vi "Error UI.vi"() -> ()   [LabVIEW 2012]
uses:
  <vilib>/Platform/TimedLoop/XDataNode/timing_clust.ctl
  <vilib>/Platform/TimedLoop/XDataNode/nitl_modes.ctl
  <vilib>/Platform/TimedLoop/XDataNode/wakeup.ctl
  <vilib>/Platform/TimedLoop/XDataNode/XDataNode.xnode
  <vilib>/Platform/TimedLoop/XDataNode/XDNodeRunTimeDep.lvlib
panel:
  out "Error":bool
  out "OK":bool
  in  "stop?":bool
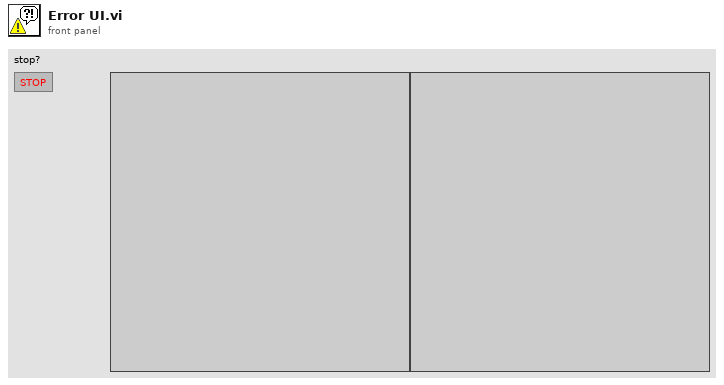
[diagram p1: front panel]
types:
  T1 = typedef "XDNodeRunTimeDep.lvlib/timing_clust.ctl" = cluster{"Expected End [f-1]":u64, "Actual End [f-1]":u64, "Finished Late? [f-1]":bool, "Expected End [i-1]":u64, "Actual End [i-1]":u64, "Finished Late? [i-1]":bool, "Expected Start [i]":u64, "Actual Start [i]":u64, "Expected Start [f]":u64, "Actual Start [f]":u64, "Source Name":string, "Structure Name":string, "Period":i64, "Deadline":i64, "Offset":i64, "Start":i64, "Priority":i32, "Timeout":i32, "Mode":T2, "Wakeup Reason":T3, "Error":errorcluster, "Source Type":string, "Secondary Source Type":string, "Global End Time":u64, "Global Start Time":u64, "Frame Duration":u64, "Iteration Duration":u64, "Assigned CPU":i32, "I/O Scan Engine Mode":u32}
  T2 = typedef "XDNodeRunTimeDep.lvlib/nitl_modes.ctl" = enum32{"No Change", "Process missed periods, maintain original phase", "Discard missed periods, maintain original phase", "Process missed periods, ignore original phase", "Discard missed periods, ignore original phase"}
  T3 = typedef "XDNodeRunTimeDep.lvlib/wakeup.ctl" = enum32{"Normal", "Aborted", "Asynchronous wakeup", "Timing source error", "Timed loop error", "Timeout"}
  T4 = enum16{"Idle", "Wiimote", "Joypad", "IGVC", "Avoide Objects", "Avoide Lines", "Path Planning", "Heading", "Waypoint"}
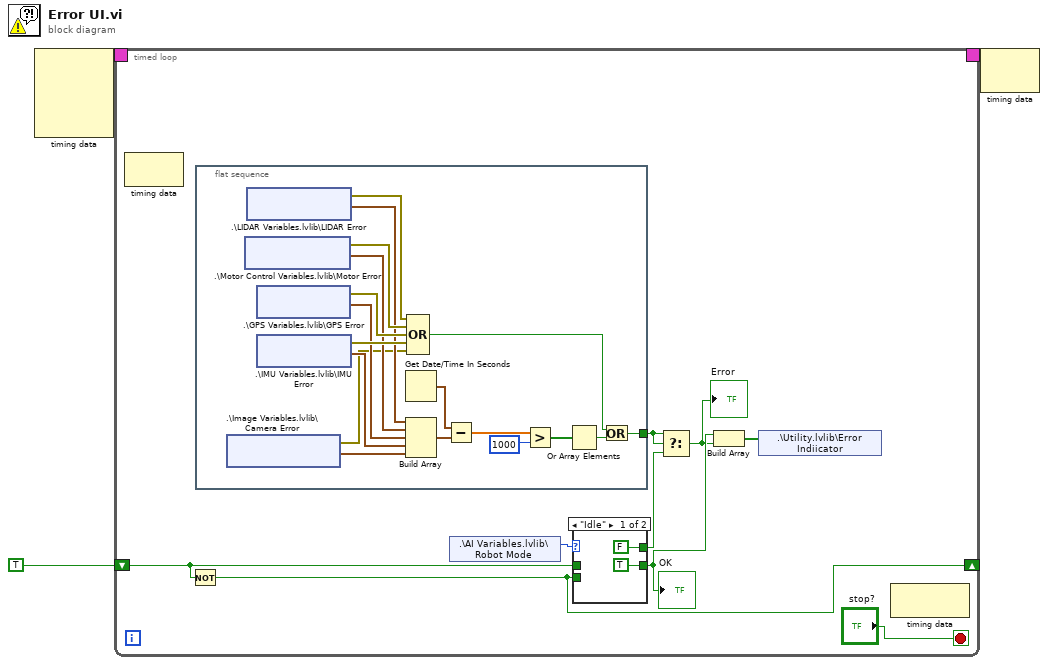
[diagram p0: block diagram]
diagram:
  n1 = node-c288() -> (w3:T1)  [unwired: 4 in]
  n2 = timed-loop {
    timing: w3 -> [_]
    timing-out: [_] -> w2
    shift-right: [w6] -> _
    shift-left: TRUE ("logical AND") -> [w8]
    stop <- "stop?" stop-if-true
    n3 = node-c288() -> ()  [unwired: 1 in, 1 out]
    n4 = Not(x=w8) -> (.not. x?=w6:bool)
    n5 = flat-sequence {
      tunnel: [w19] -> w11
      frame #0 {
        n6 = shared-variable ".\\Image Variables.lvlib\\Camera Error"() -> (w18:errorcluster, w17:timestamp)  [unwired: 1 in, 1 out]
        n7 = shared-variable ".\\Motor Control Variables.lvlib\\Motor Error"() -> (w33:errorcluster, w28:timestamp)  [unwired: 1 in, 1 out]
        n8 = shared-variable ".\\LIDAR Variables.lvlib\\LIDAR Error"() -> (w34:errorcluster, w29:timestamp)  [unwired: 1 in, 1 out]
        n9 = shared-variable ".\\GPS Variables.lvlib\\GPS Error"() -> (w32:errorcluster, w27:timestamp)  [unwired: 1 in, 1 out]
        n10 = shared-variable ".\\IMU Variables.lvlib\\IMU Error"() -> (w31:errorcluster, w26:timestamp)  [unwired: 1 in, 1 out]
        n11 = Get Date/Time In Seconds() -> (seconds since 1Jan1904=w25:timestamp)
        n12 = Build Array(w29, w28, w27, w26, w17) -> (w24:timestamp[])
        n13 = Compound Arithmetic op=OR(w34, w33, w32, w31, w18) -> (w30:bool)
        n14 = Subtract(x=w25, y=w24) -> (x-y=w23:dbl[])
        n15 = Greater?(x=w23, y=1000) -> (0:w21:bool[])
        n16 = Or Array Elements(Boolean array=w21) -> (logical OR=w20:bool)
        n17 = Or(x=w30, y=w20) -> (x .or. y?=w19:bool)
      }
    }
    n18 = shared-variable ".\\AI Variables.lvlib\\Robot Mode"() -> (w9:T4)  [unwired: 1 in, 1 out]
    n19 = case shown="\"Idle\"" w9 {
      tunnel: [TRUE ("logical AND") w16] -> w5
      tunnel: w8 -> [_ w16]
      tunnel: [FALSE w15] -> w7
      tunnel: w6 -> [_ w15]
      frame "Idle" {
      }
      frame "Wiimote", Default {
      }
    }
    "OK" <- w5
    n20 = Select(t=w11, s=w11, f=w7) -> (s? t:f=w4:bool)
    "Error" <- w4
    n21 = Build Array(w5, w4) -> (w10:bool[])
    n22 = shared-variable ".\\Utility.lvlib\\Error Indiicator"(w10) -> ()  [unwired: 1 in, 1 out]
    n23 = node-c288() -> ()  [unwired: 1 in, 1 out]
  }
  n24 = node-c288(w2) -> ()  [unwired: 1 out]
